vi "Set all f same.vi"(8 "error in (no error)":errorcluster, 11 "Instrument.DAQ":refnum<class "Instrument.DAQ.lvclass">) -> (0 "error out":errorcluster, 3 "Instrument.DAQ out":refnum<class "Instrument.DAQ.lvclass">)   [LabVIEW 2019, in "Instrument.Lockin.lvlib" / "Instrument.DAQ.lvclass"]
uses:
  Instrument.DAQ.lvclass
  Instrument.DAQ.lvclass/Instrument.DAQ.ctl
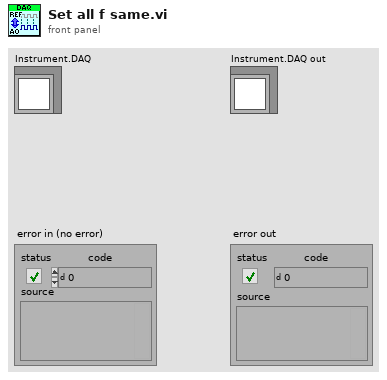
[diagram p1: front panel]
types:
  T1 = typedef "Instrument.Lockin.lvlib/Instrument.DAQ.lvclass/AO.Channel--Cluster--Array.ctl" = T2[]
  T2 = typedef "Instrument.Lockin.lvlib/Instrument.DAQ.lvclass/AO.Channel--Cluster.ctl" = cluster{"Enable?":bool, "Channel":i32, "Amplitude":dbl, "Offset":dbl, "Frequency":dbl, "Phase":dbl, "Function":T3, "Sweeping?":bool}
  T3 = typedef "Instrument.Lockin.lvlib/Instrument.DAQ.lvclass/AO.Channel.Function--Enum.ctl" = enum16{"Sine", "Triangle", "Square"}
  T4 = typedef "Instrument.Lockin.lvlib/Instrument.DAQ.lvclass/REF.Channel--Cluster--Array.ctl" = T5[]
  T5 = typedef "Instrument.Lockin.lvlib/Instrument.DAQ.lvclass/REF.Channel--Cluster.ctl" = cluster{"Enable?":bool, "Channel":i32, "Frequency":dbl, "Phase":dbl, "TC":dbl, "Roll-Off":i32}
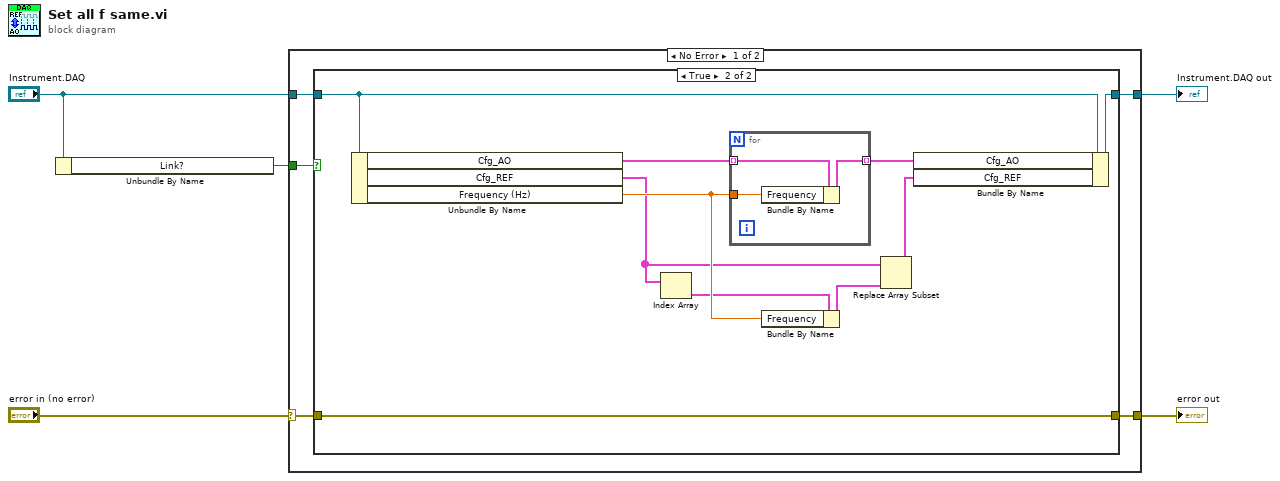
[diagram p0: block diagram]
diagram:
  n1 = Unbundle By Name("Instrument.DAQ") -> ("Link?"=w1:bool)
  n2 = case shown="No Error" "error in (no error)" {
    selector: "error in (no error)" -> [w8 w27]
    tunnel: "Instrument.DAQ" -> [w10 w26]
    tunnel: [w9 w26] -> w5
    tunnel: [w7 w27] -> w3
    tunnel: w1 -> [w6 _]
    frame No Error {
      n3 = case shown="True" w6 {
        tunnel: w10 -> [w11 w22]
        tunnel: [w11 w21] -> w9
        tunnel: w8 -> [w12 w18]
        tunnel: [w12 w18] -> w7
        frame False {
        }
        frame True {
          n4 = Unbundle By Name(w22) -> ("Cfg_AO"=w20:T1, "Cfg_REF"=w15:T4, "Frequency (Hz)"=w17:dbl)
          n5 = Index Array(array=w15) -> (element=w16:T5)  [unwired: 1 in]
          n6 = for {
            tunnel: w20 -> [w25] mode=indexing
            tunnel: [w24] -> w19 mode=indexing
            tunnel: w17 -> [w23]
            n7 = Bundle By Name(cluster=w25, "Frequency"=w23) -> (w24:T2)
          }
          n8 = Bundle By Name(cluster=w16, "Frequency"=w17) -> (w14:T5)
          n9 = Replace Array Subset(array=w15, new element=w14) -> (w13:T4)  [unwired: 1 in]
          n10 = Bundle By Name(cluster=w22, "Cfg_AO"=w19, "Cfg_REF"=w13) -> (w21:refnum<class "Instrument.DAQ.lvclass">)
        }
      }
    }
    frame Error {
    }
  }
  "error out" <- w3
  "Instrument.DAQ out" <- w5
